vi "SetCol.vi"(4 "ModeCol Index":i32=2, 5 "Col Array Ref in":refnum<vi>, 6 "Cell Position":T1, 7 "Table History ref":refnum<vi>, 8 "error in (no error)":errorcluster, 9 "Table CtlRef In":refnum<vi>, 10 "SetTo":string, 11 "ModeCol in":refnum<class "ModeCol.lvclass">) -> (0 "error out":errorcluster, 1 "Table CtlRef Out":refnum<vi>, 2 "Num Rows":i32, 3 "ModeCol out":refnum<class "ModeCol.lvclass">)   [LabVIEW 2013, in "ModeCol.lvclass"]
uses:
  ModeCol.lvclass
  <vilib>/Utility/miscctls.llb/LVRowAndColumnTypeDef.ctl
  TypeDefs/TableHistory.ctl
  TypeDefs/TableArray.ctl
  Column/Column.lvclass
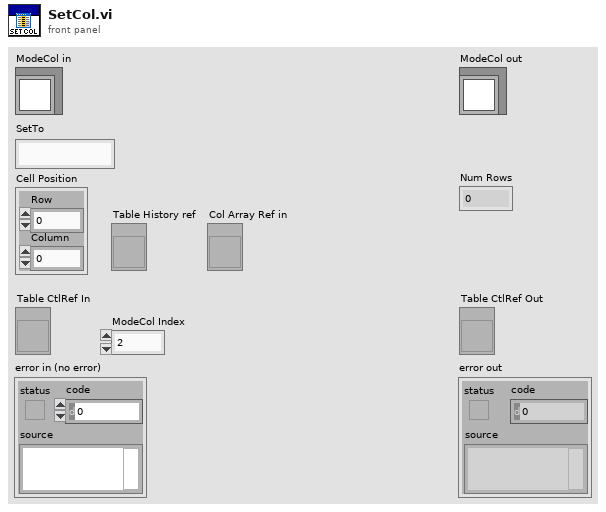
[diagram p1: front panel]
types:
  T1 = typedef "LVRowAndColumnTypeDef.ctl" = cluster{"Row":i32, "Column":i32}
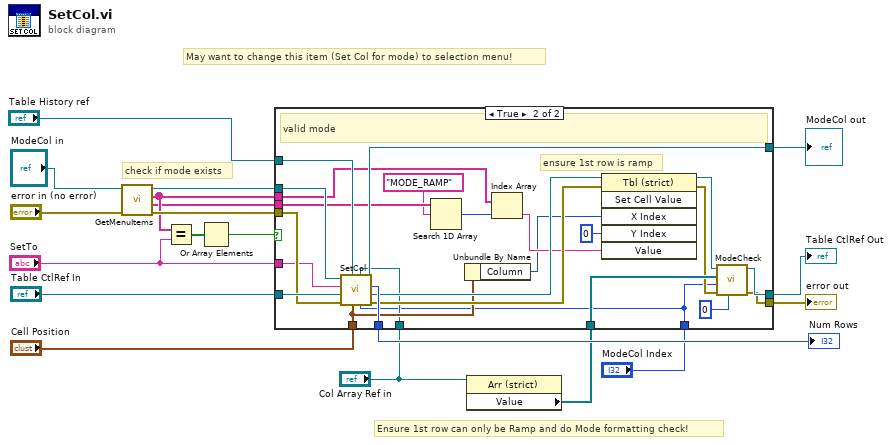
[diagram p0: block diagram]
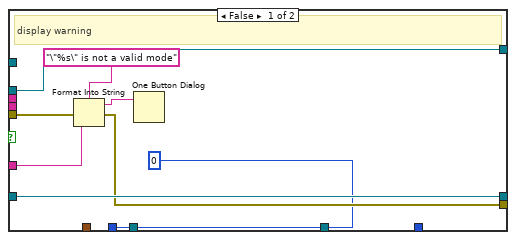
[diagram p2: hidden frame]
diagram:
  # "Ensure 1st row can only be Ramp and do Mode formatting check!"
  # "May want to change this item (Set Col for mode) to selection menu!"
  # "check if mode exists"
  n1 = call "GetMenuItems.vi"("error in (no error)"="error in (no error)", "ModeCol in"="ModeCol in") -> ("error out"=w9:errorcluster, "LMenu tags"=w4:string[], "LMenu names"=w5:string[], "ModeCol out"=w11:refnum<class "ModeCol.lvclass">)  [unwired: 6 in]
  n2 = Equal?(x=w5, y="SetTo") -> (x = y?=w7:bool[])
  n3 = Or Array Elements(Boolean array=w7) -> (logical OR=w6:bool)
  n4 = property class="Arr (strict)"(reference="Col Array Ref in") -> ("Value"=w2:refnum<class "Column.lvclass">[])  [unwired: 1 in, 2 out]
  n5 = case shown="True" w6 {
    tunnel: [w24 w42] -> w19
    tunnel: [w27 w43] -> w18
    tunnel: [0 ("Num Rows") w52] -> w17
    tunnel: [w26 w51] -> w16
    tunnel: "Cell Position" -> [_ w33]
    tunnel: "Table History ref" -> [_ w50]
    tunnel: "Table CtlRef In" -> [w27 w49]
    tunnel: w11 -> [w26 w48]
    tunnel: w9 -> [w25 w47]
    tunnel: "SetTo" -> [w23 w46]
    tunnel: w5 -> [_ w35]
    tunnel: w4 -> [_ w45]
    tunnel: "ModeCol Index" -> [_ w29]
    tunnel: w2 -> [_ w41]
    tunnel: "Col Array Ref in" -> [_ w30]
    frame False {
      # "display warning"
      n6 = Format Into String(format string="\"%s\" is not a valid mode", error in=w25, w23) -> (resulting string=w22:string, error out=w24:errorcluster)  [unwired: 1 in]
      n7 = One Button Dialog(message=w22) -> ()  [unwired: 1 in, 1 out]
    }
    frame True {
      # "ensure 1st row is ramp"
      # "valid mode"
      n8 = call-parent "SetCol.vi"("ModeCol Index"=w29, "Col Array Ref in"=w30, "Cell Position"=w33, "Table History ref"=w50, "error in (no error)"=w47, "Table CtlRef In"=w49, "SetTo"=w46, "Column in"=w48) -> ("error out"=w38:errorcluster, "Table CtlRef Out"=w40:refnum<vi>, "Num Rows"=w52:i32, "Column out"=w51:refnum<class "ModeCol.lvclass">)
      n9 = Search 1D Array(1D array=w45, element="MODE_RAMP") -> (index of element=w36:i32)  [unwired: 1 in]
      n10 = Unbundle By Name(w33) -> ("Column"=w32:i32)
      n11 = Index Array(array=w35, index=w36) -> (element=w34:string)
      n12 = invoke class="Tbl (strict)" method="Set Cell Value"(reference=w40, error in=w38, "X Index"=w32, "Y Index"=0, "Value"=w34) -> (reference out=w39:refnum<vi>, error out=w37:errorcluster)  [unwired: 1 in, 4 out]
      n13 = call "ModeCheck.vi"("Start Row (first, DISAB only)"=0 ("Start Row (first)"), "error in (no error)"=w37, "mode col. index"=w29, "Col Array in"=w41, "Table Ref in"=w39) -> ("error out"=w42:errorcluster, "Table Ref out"=w43:refnum<vi>)  [unwired: 5 in]
    }
  }
  "error out" <- w19
  "Table CtlRef Out" <- w18
  "ModeCol out" <- w16
  "Num Rows" <- w17
